vi "FRCts20_Backend_Team_PPD_reform.vi"(7 "TeamRoot":T1, 8 "error in (no error)":errorcluster, 11 "rows affected":i32) -> (0 "error out":errorcluster, 2 "data string":string)   [LabVIEW 2014, in "FRCts20_Backend_Engine.lvlib"]
doc: "Returns whether a team was successfully updated or deleted"
uses:
  FRCts20_Backend_Engine.lvlib
  FRCts20_Backend_API/Team.ctl
  FRCts20_Backend_API/ApiReturn.ctl
  FRCts20_Backend_API/TeamRoot.ctl
  FRCts20_Backend_API/FRCts20_Backend_API_SW.ctl
  FRCts20_Backend_API/TeamExtended.ctl
  FRCts20_Backend_API/EventRoot.ctl
  FRCts20_Backend_API/FRCts20_Backend_API.lvlib
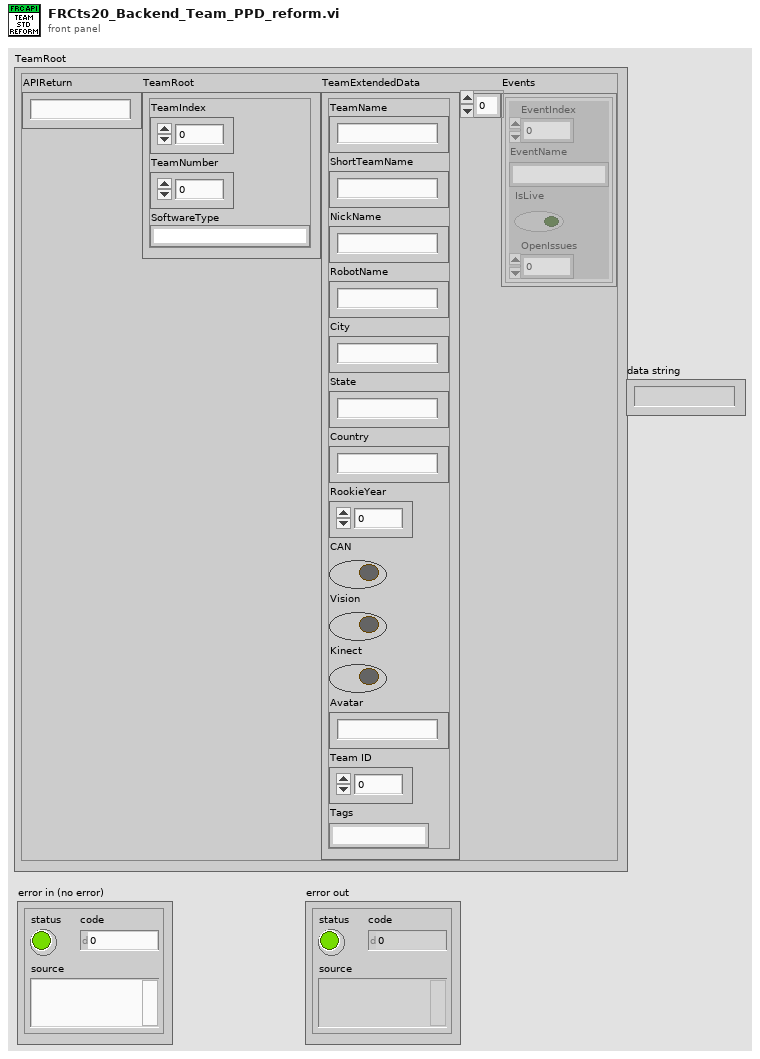
[diagram p1: front panel]
types:
  T1 = typedef "FRCts20_Backend_Engine.lvlib/FRCts20_Backend_API.lvlib/Team.ctl" = cluster{"APIReturn":T2, "TeamRoot":T3, "TeamExtendedData":T5, "Events":T6[]}
  T2 = typedef "FRCts20_Backend_Engine.lvlib/FRCts20_Backend_API.lvlib/ApiReturn.ctl" = string
  T3 = typedef "FRCts20_Backend_Engine.lvlib/FRCts20_Backend_API.lvlib/TeamRoot.ctl" = cluster{"TeamIndex":i32, "TeamNumber":u32, "SoftwareType":T4}
  T4 = typedef "FRCts20_Backend_Engine.lvlib/FRCts20_Backend_API.lvlib/FRCts20_Backend_API_SW.ctl" = string
  T5 = typedef "FRCts20_Backend_Engine.lvlib/FRCts20_Backend_API.lvlib/TeamExtended.ctl" = cluster{"TeamName":string, "ShortTeamName":string, "NickName":string, "RobotName":string, "City":string, "State":string, "Country":string, "RookieYear":u32, "CAN":bool, "Vision":bool, "Kinect":bool, "Avatar":string, "Team ID":u32, "Tags":string}
  T6 = typedef "FRCts20_Backend_Engine.lvlib/FRCts20_Backend_API.lvlib/EventRoot.ctl" = cluster{"EventIndex":i32, "EventName":string, "IsLive":bool, "OpenIssues":i32}
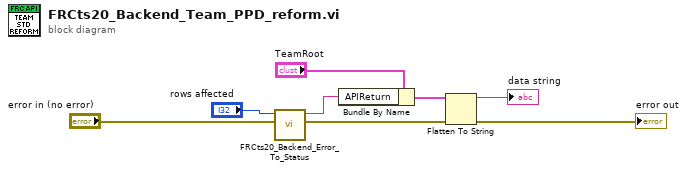
[diagram p0: block diagram]
diagram:
  n1 = call "FRCts20_Backend_Error_To_Status.vi"("error in (no error)"="error in (no error)", "rows affected"="rows affected") -> ("error out"=w4:errorcluster, "String"=w5:string)  [unwired: 8 in]
  n2 = Bundle By Name(cluster="TeamRoot", "APIReturn"=w5) -> (w1:T1)
  n3 = Flatten To String(anything=w1, error in (no error)=w4) -> (data string=→"data string":string, error out=→"error out":errorcluster)  [unwired: 2 in, 1 out]
